vi "PCAN_VERSION.vi"(7 "pathCAN_DLL":path, 8 "error in (no error)":errorcluster) -> (0 "error out":errorcluster, 2 "lpszTextBuff":string, 3 "error":T1 items=["CAN_ERR_OK"=0, "CAN_ERR_XMTFULL"=1, "CAN_ERR_OVERRUN"=2, "CAN_ERR_BUSLIGHT"=4, "CAN_ERR_BUSHEAVY"=8, "CAN_ERR_BUSOFF"=16, "CAN_ERR_QRCVEMPTY"=32, "CAN_ERR_QOVERRUN"=64, "CAN_ERR_QXMTFULL"=128, "CAN_ERR_REGTEST"=256, "CAN_ERR_NOVXD"=512, "CAN_ERR_HWINUSE"=1024, "CAN_ERR_NETINUSE"=2048, "CAN_ERR_ILLHW"=5120, "CAN_ERR_ILLNET"=6144, "CAN_ERR_ILLCLINET"=7168, "CAN_ERR_RESOURCE"=8192, "CAN_ERR_ILLPARAMTYPE"=16384, "CAN_ERR_ILLPARAMVAL"=32768, "CAN_ERR_UNKNOWN"=65536])   [LabVIEW 2023, in "pCANLib.lvlib"]
uses:
  pCANLib.lvlib
  PCAN_ERROR.ctl
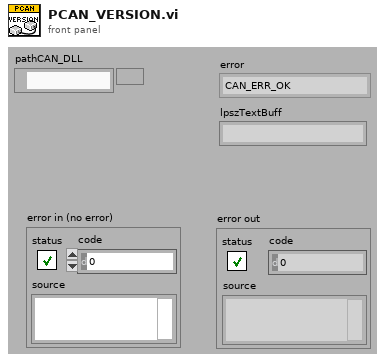
[diagram p1: front panel]
types:
  T1 = typedef "pCANLib.lvlib/PCAN_ERROR.ctl" = i32
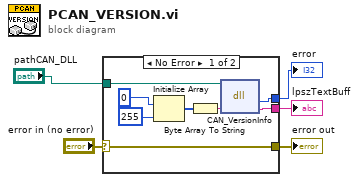
[diagram p0: block diagram]
diagram:
  n1 = case shown="No Error" "error in (no error)" {
    selector: "error in (no error)" -> [w12 w14]
    tunnel: [w13 _] -> w3
    tunnel: [w12 w14] -> w4
    tunnel: [w7 _] -> w2
    tunnel: "pathCAN_DLL" -> [w6 _]
    frame No Error {
      n2 = Initialize Array(u8 0 ("element"), 255 ("dimension size")) -> (w9:u8[])
      n3 = Byte Array To String(unsigned byte array=w9) -> (string=w8:string)
      n4 = dll-call lib="D:/PCAN/PCAN/PCAN Driver/PCAN_Driver/PCAN_USB.DLL" fn="CAN_VersionInfo"(path in=w6, "lpszTextBuff"=w8) -> ("return type"=w13:i32, "lpszTextBuff"=w7:string)  [unwired: 2 in, 2 out]
    }
    frame Error {
    }
  }
  "error out" <- w4
  "error" <- w3
  "lpszTextBuff" <- w2
